vi "fpga_Get Max.vi"(0 "previous max value":fxp<+/-,24,1>, 2 "signal in":fxp<+/-,24,1>, 3 "reset? (F)":bool) -> (4 "current max value":fxp<+/-,24,1>)   [LabVIEW 2014]
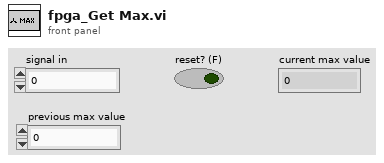
[diagram p1: front panel]
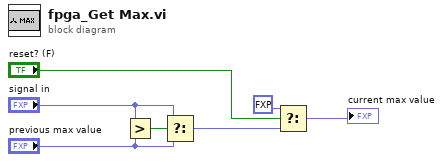
[diagram p0: block diagram]
diagram:
  n1 = Greater?(x="signal in", y="previous max value") -> (0:w7:bool)
  n2 = Select(t="signal in", s=w7, f="previous max value") -> (s? t:f=w4:fxp<+/-,24,1>)
  n3 = Select(t=fxp<+/-,24,1> 0.0 ("signal in"), s="reset? (F)", f=w4) -> (s? t:f=→"current max value":fxp<+/-,24,1>)
